vi "Write Channels' Labels.vi"(8 "error in (no error)":errorcluster, 10 "Channels' Labels":string[](array[string]), 11 "Father Of All Detectors in":refnum<class "Father Of All Detectors.lvclass">) -> (0 "error out":errorcluster, 3 "Father Of All Detectors out":refnum<class "Father Of All Detectors.lvclass">)   [LabVIEW 2026, in "TALOS.lvlib" / "Father Of All Detectors.lvlib" / "Father Of All Detectors.lvclass"]
uses:
  Father Of All Detectors.lvclass
  Father Of All Detectors.lvclass/Father Of All Detectors.ctl
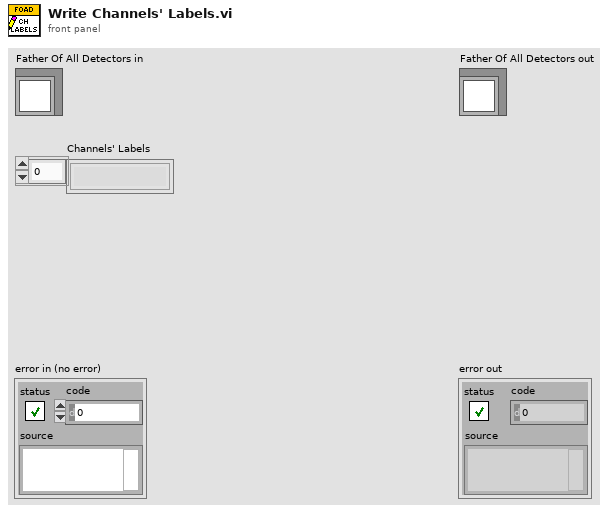
[diagram p1: front panel]
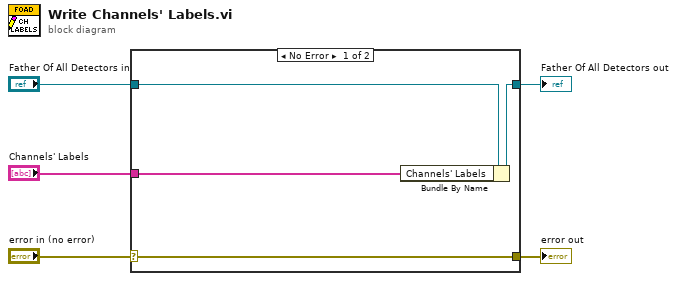
[diagram p0: block diagram]
diagram:
  n1 = case shown="No Error" "error in (no error)" {
    selector: "error in (no error)" -> [w9 w10]
    tunnel: [w9 w10] -> w4
    tunnel: [w7 w11] -> w2
    tunnel: "Father Of All Detectors in" -> [w8 w11]
    tunnel: "Channels' Labels" -> [w6 _]
    frame No Error {
      n2 = Bundle By Name(cluster=w8, "Channels' Labels"=w6) -> (w7:refnum<class "Father Of All Detectors.lvclass">)
    }
    frame Error {
    }
  }
  "error out" <- w4
  "Father Of All Detectors out" <- w2
